vi "exit.vi"() -> ()   [LabVIEW 2010]
panel:
  out "Exit":bool
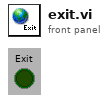
[diagram p1: front panel]
diagram:
